vi "Operand to Formula.vi"(11 "Operand":u16[](array[numeric])) -> (3 "integrand formula":string)   [LabVIEW 2023]
doc: "Generates the formula string of the integrand according to <B>Operand</B>."
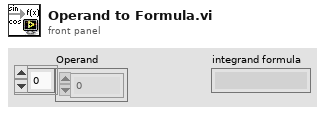
[diagram p1: front panel]
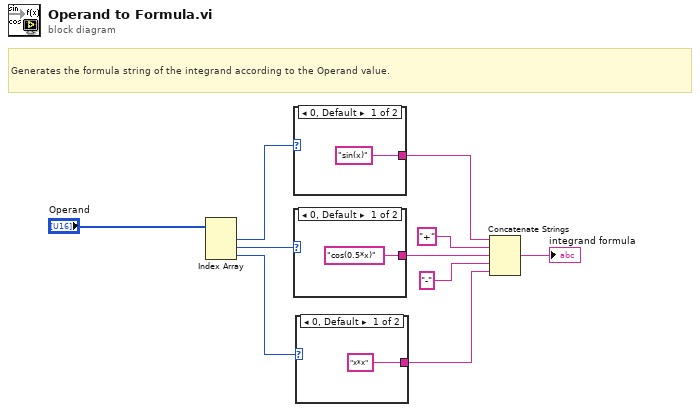
[diagram p0: block diagram]
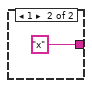
[diagram p2: hidden frame]
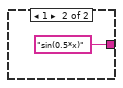
[diagram p3: hidden frame]
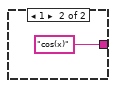
[diagram p4: hidden frame]
diagram:
  # "Generates the formula string of the integrand according to the Operand value."
  n1 = Index Array(array="Operand") -> (element #1=w9:u16, element #2=w8:u16, element #3=w7:u16)  [unwired: 3 in]
  n2 = case shown="0, Default" w9 {
    tunnel: ["sin(x)" "cos(x)"] -> w6
    frame 0, Default {
    }
    frame 1 {
    }
  }
  n3 = case shown="0, Default" w8 {
    tunnel: ["cos(0.5*x)" "sin(0.5*x)"] -> w5
    frame 0, Default {
    }
    frame 1 {
    }
  }
  n4 = case shown="0, Default" w7 {
    tunnel: ["x*x" "x"] -> w4
    frame 0, Default {
    }
    frame 1 {
    }
  }
  n5 = Concatenate Strings(w6, "+", w5, "-", w4) -> (→"integrand formula":string)
